vi "Remove PUBREC.vi"(8 "error in (no error)":errorcluster, 10 "Packet Identifier":u16 format="%016b", 11 "Client ID":string) -> (0 "error out":errorcluster)   [LabVIEW 2013, in "MQTT Server.lvlib" / "StoredSessions.lvclass"]
uses:
  StoredSessions.lvclass
  Session State -- cluster.ctl
  <vilib>/LabVIEW Open Source Project/MQTT Control Packets/Control Packets/SUBSCRIBE/Topic Subscription -- cluster.ctl
  <vilib>/LabVIEW Open Source Project/MQTT Control Packets/Control Packets/ControlPacket/QualityOfService -- enum.ctl
  <vilib>/LabVIEW Open Source Project/MQTT Control Packets/Control Packets/ControlPacket/ControlPacket.lvclass
  <vilib>/LabVIEW Open Source Project/MQTT Control Packets/Control Packets/SUBSCRIBE/SUBSCRIBE.lvclass
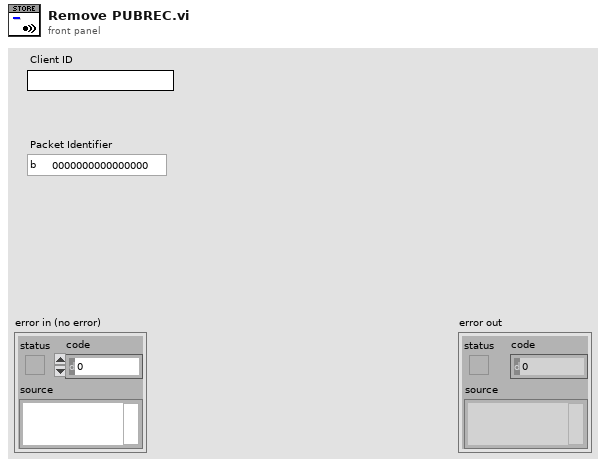
[diagram p1: front panel]
types:
  T1 = typedef "MQTT Server.lvlib/StoredSessions.lvclass/Session State -- cluster.ctl" = cluster{"Client ID":string, "Subscriptions":T2[], "PUBREC":u16[]}
  T2 = typedef "MQTT_Control_Packets.lvlib/SUBSCRIBE.lvclass/Topic Subscription -- cluster.ctl" = cluster{"Topic Filter":string, "QoS":T3}
  T3 = typedef "MQTT_Control_Packets.lvlib/ControlPacket.lvclass/QualityOfService -- enum.ctl" = enum16{"0 (At Most Once)", "1 (At Least Once)", "2 (Exactly Once)"}
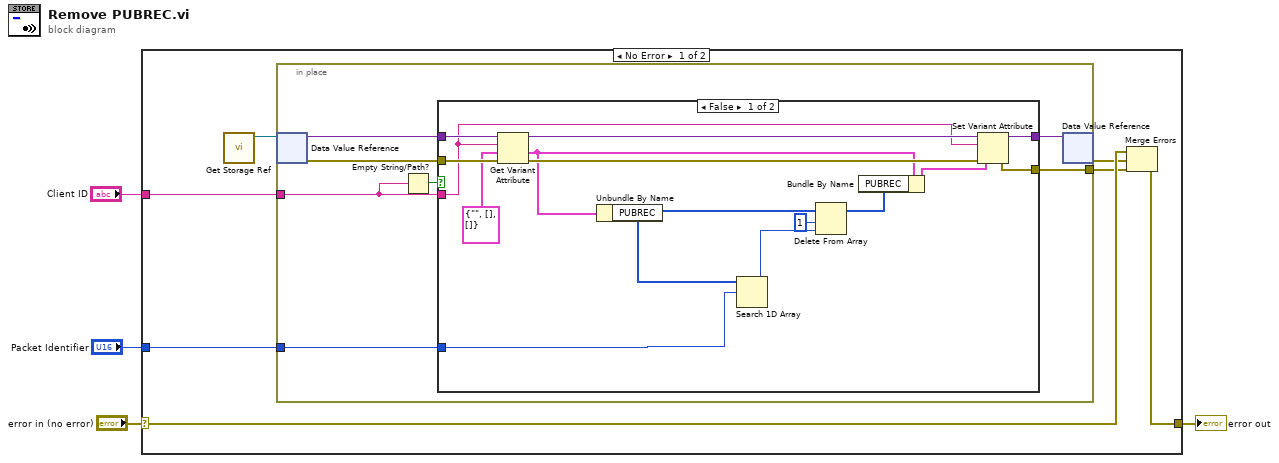
[diagram p0: block diagram]
diagram:
  n1 = case shown="No Error" "error in (no error)" {
    selector: "error in (no error)" -> [w11 w36]
    tunnel: [w10 w36] -> w3
    tunnel: "Packet Identifier" -> [w9 _]
    tunnel: "Client ID" -> [w8 _]
    frame No Error {
      n2 = call "Get Storage Ref.vi"() -> ("Storage"=w7:refnum<data-value>)  [unwired: 11 in]
      n3 = in-place {
        in-place-border: w9 -> [w12]
        in-place-border: [w16] -> w5
        in-place-border: w8 -> [w13]
        n4 = in-place-dvr #1(w7) -> (w18:variant, w15:errorcluster)
        n5 = Empty String/Path?(string/path=w13) -> (empty?=w14:bool)
        n6 = case shown="False" w14 {
          tunnel: w18 -> [w33 w35]
          tunnel: [w30 w35] -> w17
          tunnel: [w21 w34] -> w16
          tunnel: w15 -> [w32 w34]
          tunnel: w13 -> [w27 _]
          tunnel: w12 -> [w20 _]
          frame False {
            n7 = Get Variant Attribute(Variant=w33, name=w27, default value (empty Variant)=T1 {"Client ID"="", "Subscriptions"=[], "PUBREC"=[]} ("Stored Session"), error in=w32) -> (duplicate Variant=w31:variant, value=w26:T1, error out=w28:errorcluster)  [unwired: 1 out]
            n8 = Unbundle By Name(w26) -> ("PUBREC"=w19:u16[])
            n9 = Search 1D Array(1D array=w19, element=w20) -> (index of element=w23:i32)  [unwired: 1 in]
            n10 = Delete From Array(array=w19, length=1, index=w23) -> (array with subset deleted=w24:u16[])  [unwired: 1 out]
            n11 = Bundle By Name(cluster=w26, "PUBREC"=w24) -> (w25:T1)
            n12 = Set Variant Attribute(Variant=w31, name=w27, value=w25, error in=w28) -> (Variant out=w30:variant, error out=w21:errorcluster)  [unwired: 1 out]
          }
          frame True {
          }
        }
        n13 = in-place-dvr #1(w17) -> (w6:errorcluster)  [unwired: 1 out]
      }
      n14 = Merge Errors(w11, w6, w5) -> (w10:errorcluster)
    }
    frame Error {
    }
  }
  "error out" <- w3
